vi "打开文件.vi"(8 "error in (no error)":errorcluster caption="错误输入（无错误）", 11 "配置文件- 输入":refnum<class "配置文件-.lvclass">) -> (0 "error out":errorcluster caption="错误输出", 3 "配置文件- 输出":refnum<class "配置文件-.lvclass">)   [LabVIEW 2017, in "项目开发助手.lvlib" / "模板-配置文件相关.lvlib" / "配置文件-.lvclass"]
uses:
  <vilib>/Utility/config.llb/NI_LVConfig.lvlib
panel:
  in  "配置文件路径":path caption="配置文件的路径"
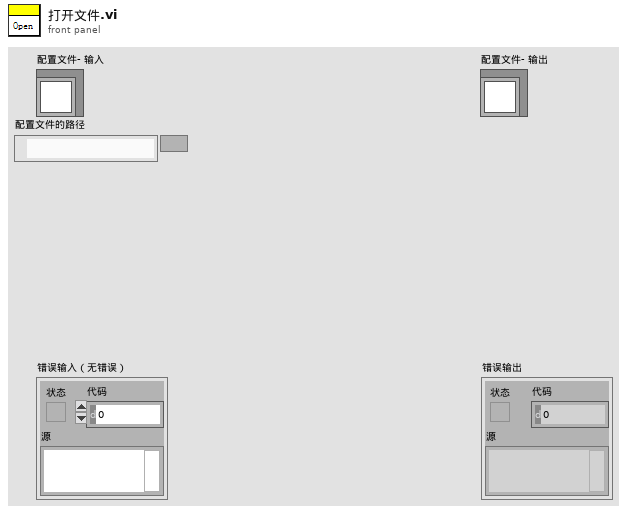
[diagram p1: front panel]
types:
  T1 = typedef "NI_LVConfig.lvlib/Config Data RefNum.ctl" = refnum<k1>
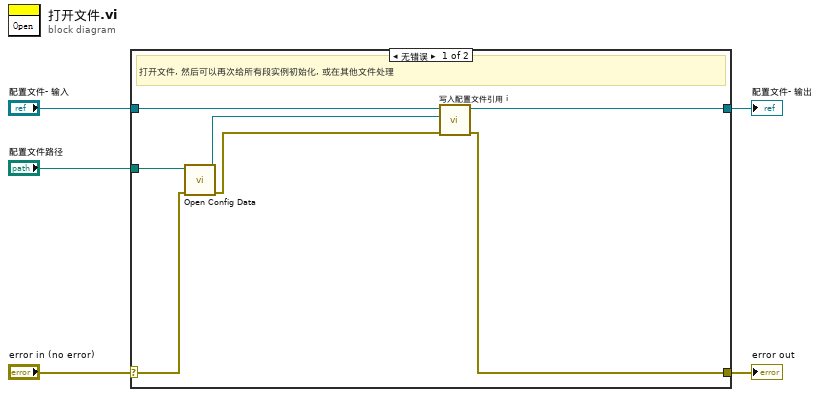
[diagram p0: block diagram]
diagram:
  n1 = case shown="无错误" "error in (no error)" {
    selector: "error in (no error)" -> [w10 w14]
    tunnel: [w6 w14] -> w4
    tunnel: [w9 w13] -> w2
    tunnel: "配置文件- 输入" -> [w12 w13]
    tunnel: "配置文件路径" -> [w11 _]
    frame No Error {
      # "打开文件, 然后可以再次给所有段实例初始化, 或在其他文件处理"
      n2 = call <vilib>:"Open Config Data.vi"("error in (no error)"=w10, "configuration file path"=w11) -> ("error out"=w7:errorcluster, "refnum"=w8:T1)  [unwired: 7 in, 1 out]
      n3 = call "写入配置文件引用 i.vi"("error in (no error)"=w7, "config data"=w8, "配置文件-输入"=w12) -> ("error out"=w6:errorcluster, "配置文件-输出"=w9:refnum<class "配置文件-.lvclass">)  [unwired: 7 in]
    }
    frame Error {
    }
  }
  "error out" <- w4
  "配置文件- 输出" <- w2
